vi "VISARead.vi"(5 "Delete Termination Char (False)":bool, 7 "Termination Char (blank)":string, 8 "error in (no error)":errorcluster, 9 "Timeout (ms)":u32, 10 "Byte to Read (0)":u32, 11 "Resource in":refnum<visa-resource-name>) -> (0 "error out":errorcluster, 2 "Read Char":string, 3 "Resource out":refnum<visa-resource-name>)   [LabVIEW 2020, in "Reader.lvlib"]
doc: "Reads from serial port."
uses:
  UART/Reader.lvlib
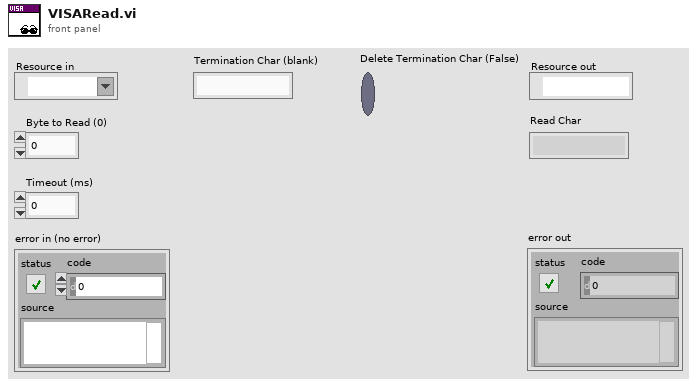
[diagram p1: front panel]
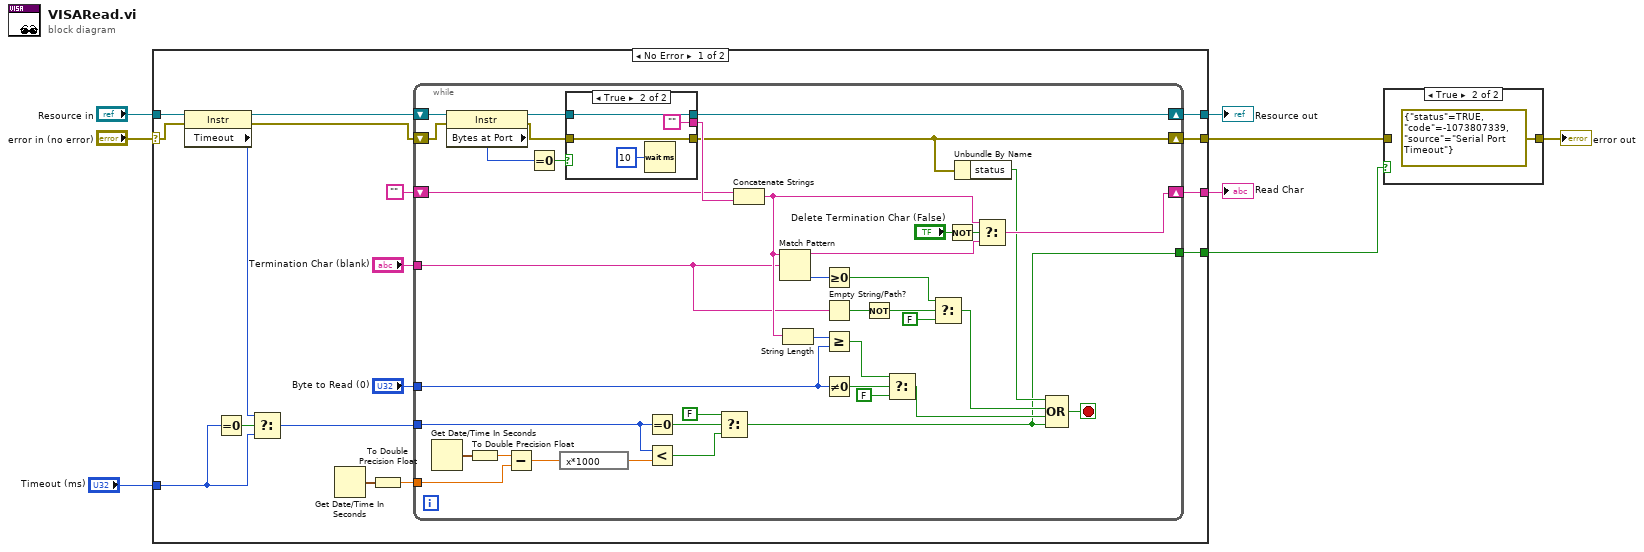
[diagram p0: block diagram]
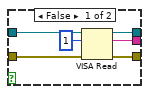
[diagram p3: hidden frame]
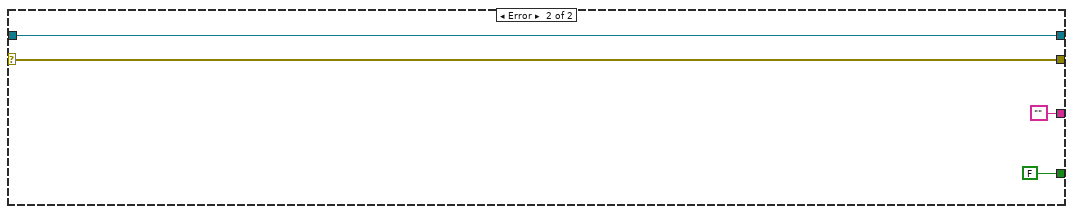
[diagram p4: hidden frame]
diagram:
  n1 = case shown="No Error" "error in (no error)" {
    selector: "error in (no error)" -> [w21 w78]
    tunnel: "Resource in" -> [w25 w79]
    tunnel: [w14 w79] -> w6
    tunnel: [w13 w78] -> w3
    tunnel: [w12 ""] -> w5
    tunnel: [w11 FALSE ("t")] -> w4
    tunnel: "Timeout (ms)" -> [w9 _]
    frame No Error {
      n2 = property class="Instr"(reference=w25, error in=w21) -> (reference out=w22:refnum<visa-resource-name>, error out=w20:errorcluster, "Timeout"=w23:u32)
      n3 = Equal To 0?(x=w9) -> (x = 0?=w24:bool)
      n4 = Select(t=w23, s=w24, f=w9) -> (s? t:f=w10:u32)
      n5 = Get Date/Time In Seconds() -> (seconds since 1Jan1904=w17:timestamp)
      n6 = To Double Precision Float(number=w17) -> (double precision float=w16:dbl)
      n7 = while {
        shift-right: [w34] -> w13
        shift-left: w20 -> [w64]
        shift-right: [w60] -> w14
        shift-left: w22 -> [w65]
        shift-right: [w54] -> w12
        shift-left: "" -> [w57]
        tunnel: w10 -> [w49]
        tunnel: "Termination Char (blank)" -> [w37]
        tunnel: w16 -> [w50]
        tunnel: "Byte to Read (0)" -> [w43]
        tunnel: [w31] -> w11
        stop <- w32 stop-if-true
        n8 = Get Date/Time In Seconds() -> (seconds since 1Jan1904=w52:timestamp)
        n9 = property class="Instr"(reference=w65, error in=w64) -> (reference out=w61:refnum<visa-resource-name>, error out=w59:errorcluster, "Bytes at Port"=w63:u32)
        n10 = To Double Precision Float(number=w52) -> (double precision float=w51:dbl)
        n11 = Subtract(x=w51, y=w50) -> (x-y=w26:dbl)
        n12 = Equal To 0?(x=w63) -> (x = 0?=w62:bool)
        n13 = expression code="x*1000"(w26) -> (w27:dbl)
        n14 = case shown="True" w62 {
          tunnel: w61 -> [w69 w75]
          tunnel: [w70 w75] -> w60
          tunnel: [w71 ""] -> w58
          tunnel: w59 -> [w67 w74]
          tunnel: [w66 w74] -> w34
          frame False {
            n15 = VISA Read(VISA resource name=w69, byte count=u32 1, error in (no error)=w67) -> (VISA resource name out=w70:refnum<visa-resource-name>, read buffer=w71:string, error out=w66:errorcluster)  [unwired: 1 out]
          }
          frame True {
            n16 = Wait (ms)(milliseconds to wait=u32 10) -> ()  [unwired: 1 out]
          }
        }
        n17 = Equal To 0?(x=w49) -> (x = 0?=w48:bool)
        n18 = Less?(x=w49, y=w27) -> (x < y?=w47:bool)
        n19 = Select(t=FALSE, s=w48, f=w47) -> (s? t:f=w31:bool)
        n20 = Concatenate Strings(w57, w58) -> (w45:string)
        n21 = Match Pattern(string=w45, regular expression=w37) -> (before substring=w53:string, offset past match=w38:i32)  [unwired: 3 out]
        n22 = String Length(string=w45) -> (length=w44:i32)
        n23 = Greater Or Equal To 0?(x=w38) -> (x >= 0?=w28:bool)
        n24 = Empty String/Path?(string/path=w37) -> (empty?=w36:bool)
        n25 = Greater Or Equal?(x=w44, y=w43) -> (x >= y?=w41:bool)
        n26 = Not Equal To 0?(x=w43) -> (x != 0?=w42:bool)
        n27 = Not(x=w36) -> (.not. x?=w29:bool)
        n28 = Select(t=w41, s=w42, f=FALSE) -> (s? t:f=w39:bool)
        n29 = Select(t=w28, s=w29, f=FALSE ("empty?")) -> (s? t:f=w35:bool)
        n30 = Not(x="Delete Termination Char (False)") -> (.not. x?=w55:bool)
        n31 = Unbundle By Name(w34) -> ("status"=w33:bool)
        n32 = Select(t=w45, s=w55, f=w53) -> (s? t:f=w54:string)
        n33 = Compound Arithmetic op=OR(w33, w35, w39, w31) -> (w32:bool)
      }
    }
    frame Error {
    }
  }
  "Resource out" <- w6
  "Read Char" <- w5
  n34 = case shown="True" w4 {
    tunnel: w3 -> [w80 _]
    tunnel: [w80 errorcluster {"status"=TRUE, "code"=-1073807339, "source"="Serial Port Timeout"} ("error IO")] -> w2
    frame False {
    }
    frame True {
    }
  }
  "error out" <- w2
